vi "iteraciones.vi"() -> ()   [LabVIEW 2020]
panel:
  out "Iteracion":dbl
  in  "Numeric 2":i32
  out "=":dbl
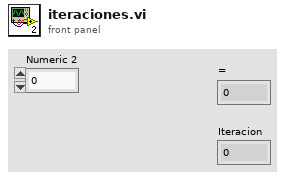
[diagram p1: front panel]
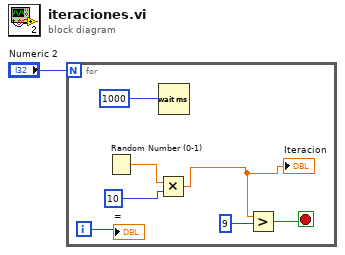
[diagram p0: block diagram]
diagram:
  n1 = for {
    N: "Numeric 2" -> [_]
    i -> [w3]
    stop <- w5 stop-if-true
    n2 = Random Number (0-1)() -> (number: 0 to 1=w8:dbl)
    n3 = Multiply(x=w8, y=10) -> (x*y=w2:dbl)
    "Iteracion" <- w2
    n4 = Wait (ms)(milliseconds to wait=1000) -> ()  [unwired: 1 out]
    n5 = Greater?(x=w2, y=9) -> (0:w5:bool)
    "=" <- w3
  }
